vi "Configure VST.vi"(8 "error in (no error)":errorcluster, 10 "VST Config":T1={"Samples to Read per Block"=33554432, "IQ rate (S/s)"=1250000000.0, "Carrier Frequency (Hz)"=1000000000.0, "Reference Level (dBm)"=0.0, "Resource Name"="RFSA", "Clock Source"="OnboardClock", "Host DMA Buffer Size"=2000000000} {"Host DMA Buffer Size" format="%.0p"; "Reference Level (dBm)" format="%.2f"; "Carrier Frequency (Hz)" format="%#.3p"; "IQ rate (S/s)" format="%#.3p"; "Samples to Read per Block" min=1 format="%.0p"}, 11 "RFSA DAQ in":refnum<class "RFSA DAQ.lvclass">) -> (0 "error out":errorcluster, 3 "RFSA DAQ out":refnum<class "RFSA DAQ.lvclass">)   [LabVIEW 2020, in "RFSA DAQ.lvlib" / "RFSA DAQ.lvclass"]
uses:
  RFSA DAQ.lvclass
  Configure VST.ctl
  Helper Loop Message.ctl
  Helper Loop Type.ctl
  RFSA DAQ.lvclass/RFSA DAQ.ctl
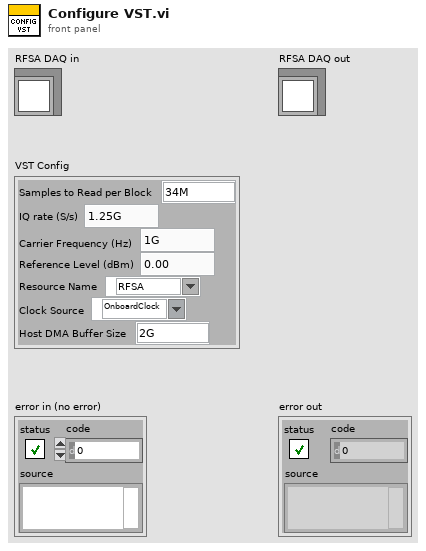
[diagram p1: front panel]
types:
  T1 = typedef "RFSA DAQ.lvlib/RFSA DAQ.lvclass/Configure VST.ctl" = cluster{"Samples to Read per Block":i32, "IQ rate (S/s)":dbl, "Carrier Frequency (Hz)":dbl, "Reference Level (dBm)":dbl, "Resource Name":refnum<k15>, "Clock Source":refnum<k15>, "Host DMA Buffer Size":i64}
  T2 = typedef "RFSA DAQ.lvlib/RFSA DAQ.lvclass/Helper Loop Message.ctl" = cluster{"Type":T3, "Payload":variant}
  T3 = typedef "RFSA DAQ.lvlib/RFSA DAQ.lvclass/Helper Loop Type.ctl" = enum16{"Configure", "Start", "Do", "Stop", "Clean", "Close"}
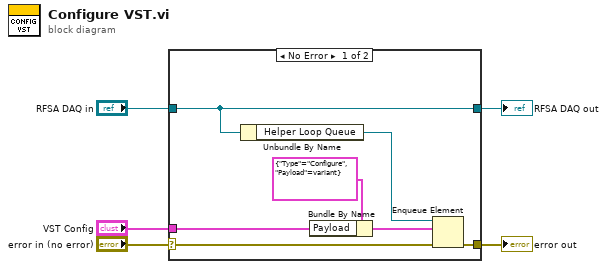
[diagram p0: block diagram]
diagram:
  n1 = case shown="No Error" "error in (no error)" {
    selector: "error in (no error)" -> [w10 w14]
    tunnel: [w8 w14] -> w4
    tunnel: [w9 w13] -> w2
    tunnel: "RFSA DAQ in" -> [w9 w13]
    tunnel: "VST Config" -> [w6 _]
    frame No Error {
      n2 = Unbundle By Name(w9) -> ("Helper Loop Queue"=w12:refnum<queue>)
      n3 = Bundle By Name(cluster=T2 {"Type"=enum."Configure", "Payload"=variant} ("element"), "Payload"=w6) -> (w7:T2)
      n4 = Enqueue Element(queue=w12, element=w7, error in (no error)=w10) -> (error out=w8:errorcluster)  [unwired: 1 in, 2 out]
    }
    frame Error {
    }
  }
  "error out" <- w4
  "RFSA DAQ out" <- w2
